vi "dB calculation with  Pmin and Pmax.vi"() -> ()   [LabVIEW 2014]
panel:
  out "x*y":dbl
  in  "0 dB volts":dbl=0.8 format="%#_13g"
  in  "volts":dbl=0.5 format="%#_13g"
  in  "Pmax":dbl=60.0
  in  "Pmin":dbl=40.0
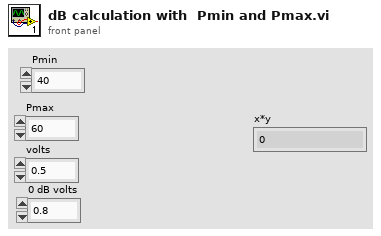
[diagram p1: front panel]
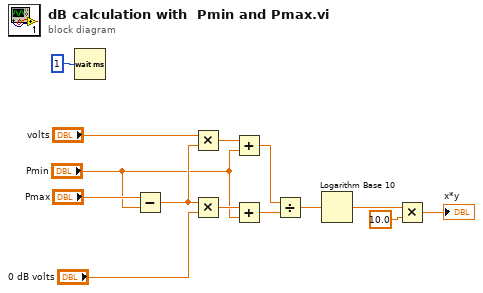
[diagram p0: block diagram]
diagram:
  n1 = Wait (ms)(milliseconds to wait=u32 1) -> ()  [unwired: 1 out]
  n2 = Subtract(x="Pmax", y="Pmin") -> (x-y=w8:dbl)
  n3 = Multiply(x="volts", y=w8) -> (x*y=w10:dbl)
  n4 = Multiply(x=w8, y="0 dB volts") -> (x*y=w6:dbl)
  n5 = Add(x=w10, y="Pmin") -> (x+y=w9:dbl)
  n6 = Add(x=w6, y="Pmin") -> (x+y=w4:dbl)
  n7 = Divide(x=w9, y=w4) -> (x/y=w3:dbl)
  n8 = Logarithm Base 10(1:w3) -> (0:w14:dbl)
  n9 = Multiply(x=w14, y=10.0) -> (x*y=→"x*y":dbl)
